vi "macaddress.vi"(10 "source MAC address":u8[](array[numeric])) -> (0 "MAC Address HEX":string, 3 "MAC Address":string)   [LabVIEW 2017]
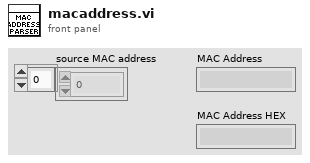
[diagram p1: front panel]
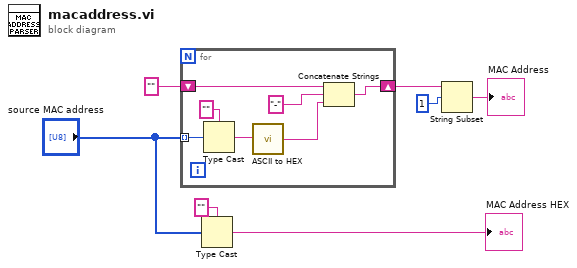
[diagram p0: block diagram]
diagram:
  n1 = for {
    tunnel: "source MAC address" -> [w14] mode=indexing
    shift-right: [w10] -> w3
    shift-left: "" -> [w9]
    n2 = Type Cast(type="", x=w14) -> (*(type *) &x=w12:string)
    n3 = call "ASCII to HEX.vi"("String in ASCII"=w12) -> ("String in HEX"=w8:string)
    n4 = Concatenate Strings(w9, "-" ("string"), w8) -> (w10:string)
  }
  n5 = Type Cast(type="", x="source MAC address") -> (*(type *) &x=→"MAC Address HEX":string)
  n6 = String Subset(string=w3, offset (0)=1) -> (substring=→"MAC Address":string)  [unwired: 1 in]
